vi "TCP_SEND_WAVEFORM.vi"(2 "error in (no error)":errorcluster, 3 "connection ID":refnum<k5>, 4 "waveform":waveform(dbl)) -> (0 "error out":errorcluster, 1 "connection ID out":refnum<k5>)   [LabVIEW 2023]
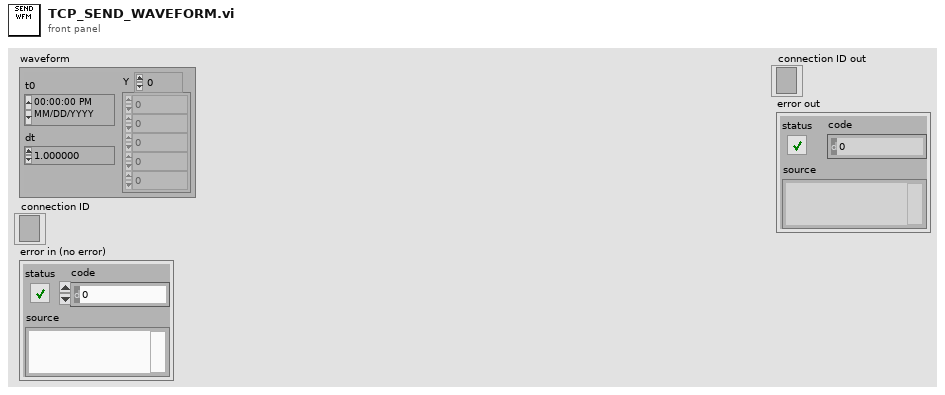
[diagram p1: front panel]
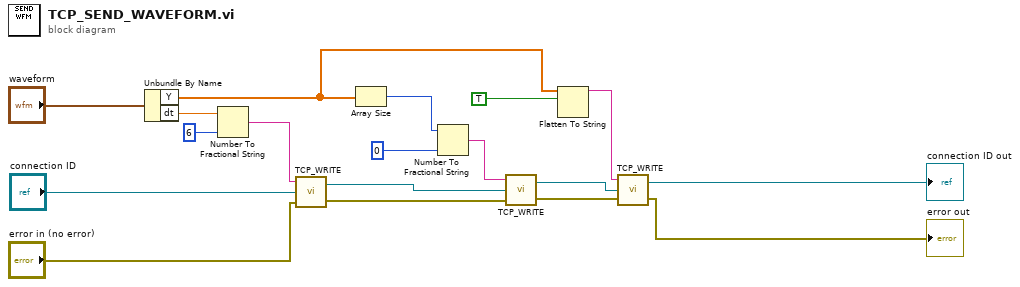
[diagram p0: block diagram]
diagram:
  n1 = Unbundle By Name("waveform") -> ("Y"=w2:dbl[], "dt"=w15:dbl)
  n2 = Number To Fractional String(number=w15, precision (6)=i16 6) -> (F-format string=w13:string)  [unwired: 2 in]
  n3 = call "TCP_WRITE.vi"("error in (no error)"="error in (no error)", "connection ID"="connection ID", "data"=w13) -> ("error out"=w11:errorcluster, "connection ID out"=w12:refnum<k5>)
  n4 = Array Size(array=w2) -> (size(s)=w10:i32)
  n5 = Number To Fractional String(number=w10, precision (6)=i16 0) -> (F-format string=w8:string)  [unwired: 2 in]
  n6 = call "TCP_WRITE.vi"("error in (no error)"=w11, "connection ID"=w12, "data"=w8) -> ("error out"=w6:errorcluster, "connection ID out"=w7:refnum<k5>)
  n7 = Flatten To String(anything=w2, prepend array or string size? (T)=TRUE) -> (data string=w3:string)  [unwired: 2 in, 2 out]
  n8 = call "TCP_WRITE.vi"("error in (no error)"=w6, "connection ID"=w7, "data"=w3) -> ("error out"=→"error out":errorcluster, "connection ID out"=→"connection ID out":refnum<k5>)
